vi "Exit.vi"(8 "error in":errorcluster, 9 "Message Sin":refnum<queue>, 10 "Message Acq":refnum<queue>, 11 "Message Cam":refnum<queue>) -> (0 "error out":errorcluster)   [LabVIEW 2020]
uses:
  SuportVI2/Message Queue/Message Cluster.ctl
  SuportVI2/Message Queue/Message Queue.lvlib
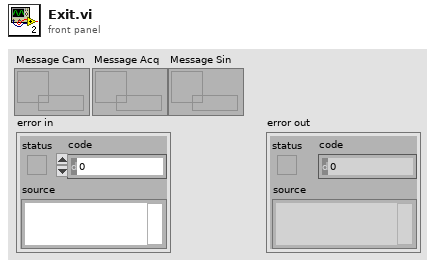
[diagram p1: front panel]
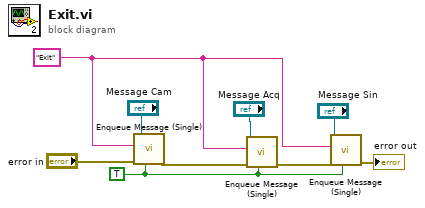
[diagram p0: block diagram]
diagram:
  w1 = TRUE ("Priority Message? (F)")
  w4 = "Exit" ("Message")
  n1 = call "Enqueue Message (Single).vi"("Priority Message? (F)"=w1, "error in (no error)"="error in", "Message"=w4, "Message Queue"="Message Cam") -> ("error out"=w6:errorcluster)  [unwired: 6 in, 1 out]
  n2 = call "Enqueue Message (Single).vi"("Priority Message? (F)"=w1, "error in (no error)"=w6, "Message"=w4, "Message Queue"="Message Acq") -> ("error out"=w3:errorcluster)  [unwired: 6 in, 1 out]
  n3 = call "Enqueue Message (Single).vi"("Priority Message? (F)"=w1, "error in (no error)"=w3, "Message"=w4, "Message Queue"="Message Sin") -> ("error out"=→"error out":errorcluster)  [unwired: 6 in, 1 out]
